vi "Example2.vi"() -> ()   [LabVIEW 2020]
doc: "Pressents differnce between type def and strict type def."
uses:
  Ctrl/Numeric2.ctl
  Ctrl/Numeric1.ctl
panel:
  in  "Numeric 1":T1
  in  "Numeric 2 Test":T2 format="%.2f"
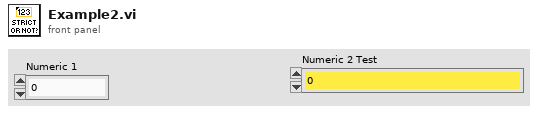
[diagram p1: front panel]
types:
  T1 = typedef "Numeric1.ctl" = i32
  T2 = typedef "Numeric2.ctl" = i32
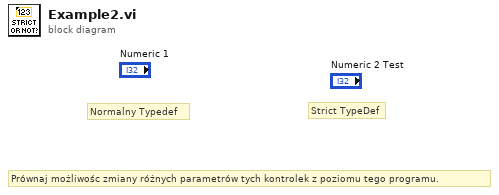
[diagram p0: block diagram]
diagram:
  # "Prównaj możliwośc zmiany różnych parametrów tych kontrolek z poziomu tego programu."
  # "Strict TypeDef"
  # "Normalny Typedef"
